vi "adc_avg.vi"(0 "CCS":T1={"Port Number"=1444, "Core Number"=1, "Page"=0}, 11 "error in":errorcluster) -> (4 "CCS out":T1={"Port Number"=1444, "Core Number"=1, "Page"=0})   [LabVIEW 2019]
uses:
  <userlib>/_TI-LA/Reusable/CCS/APIs/Data/Polymorphics/Write Data To Symbol - U16.vi
  <userlib>/_TI-LA/Reusable/CCS/APIs/Data/Polymorphics/Read Data From Symbol - U16 Array.vi
  <vilib>/Utility/file.llb/Write Delimited Spreadsheet (DBL).vi
  <vilib>/Utility/file.llb/Write Delimited Spreadsheet (I64).vi
  <userlib>/_TI-LA/Reusable/CCS/APIs/CCS.lvlib
panel:
  out "size(s)":i32
  out "x/y":dbl[](array[numeric])
  out "Array":i32[](array[numeric])
  out "error out":errorcluster
  # "uint16_t lv_ref_sel     =   0; //0=vdda, 1=extref, 2=intref\nuint16_t lv_ref_vol     =   0; //0=2P5V, 1=1P4V\nuint16_t lv_scomp       =   8; //8Clocks of 32M give = 250ns"
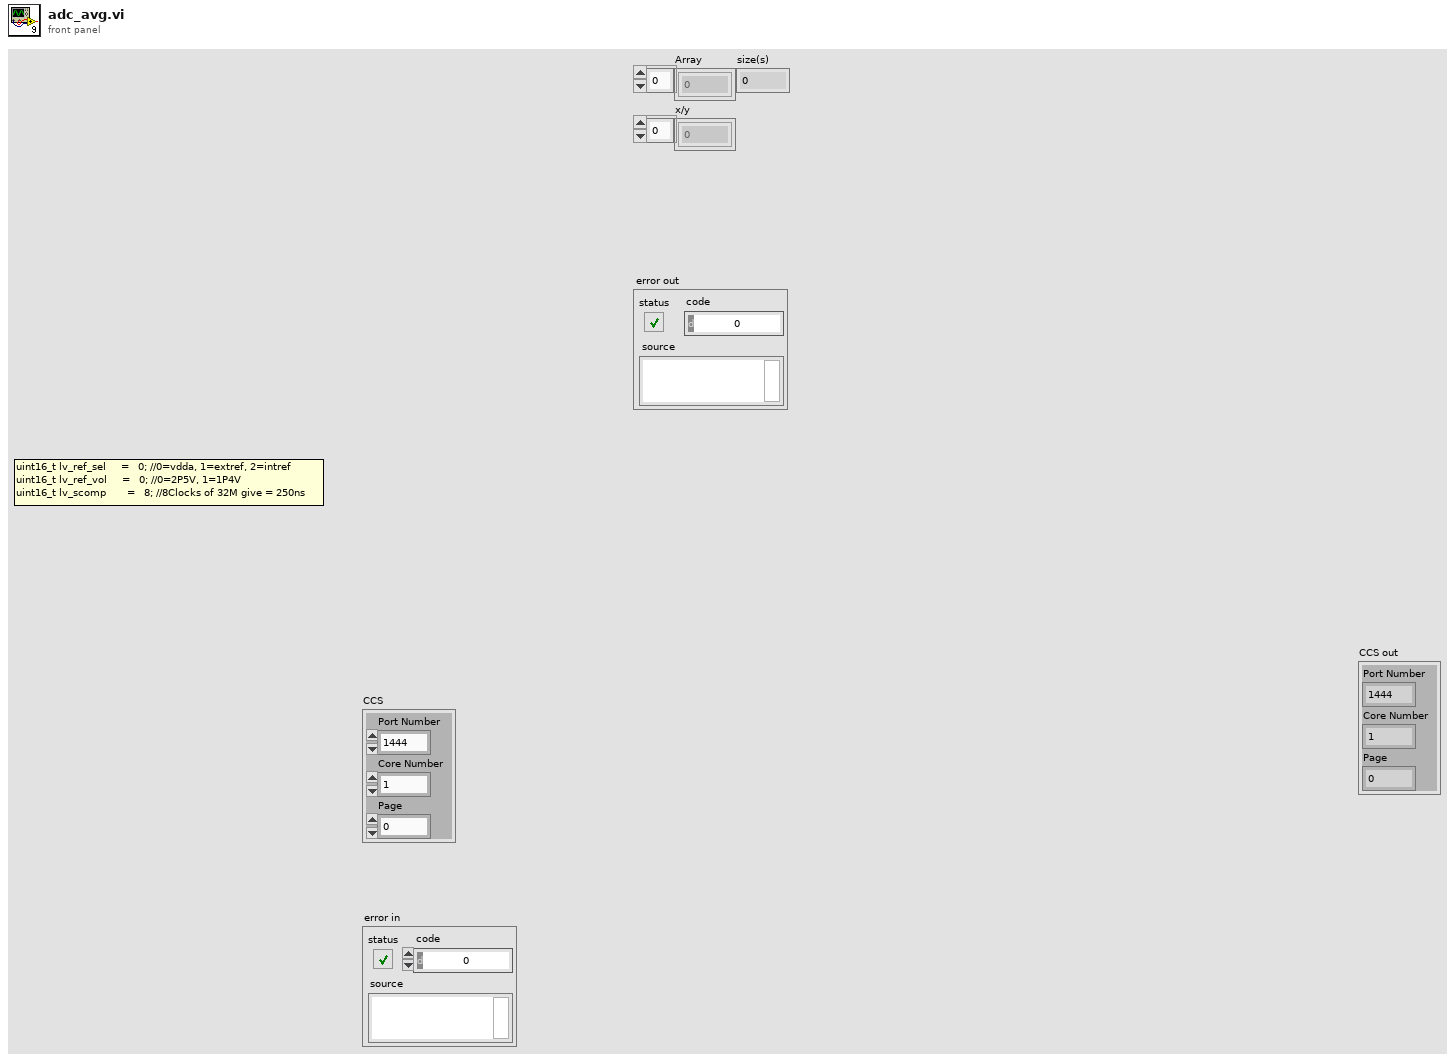
[diagram p1: front panel]
types:
  T1 = cluster{"Port Number":u16, "Core Number":u16, "Page":i32}
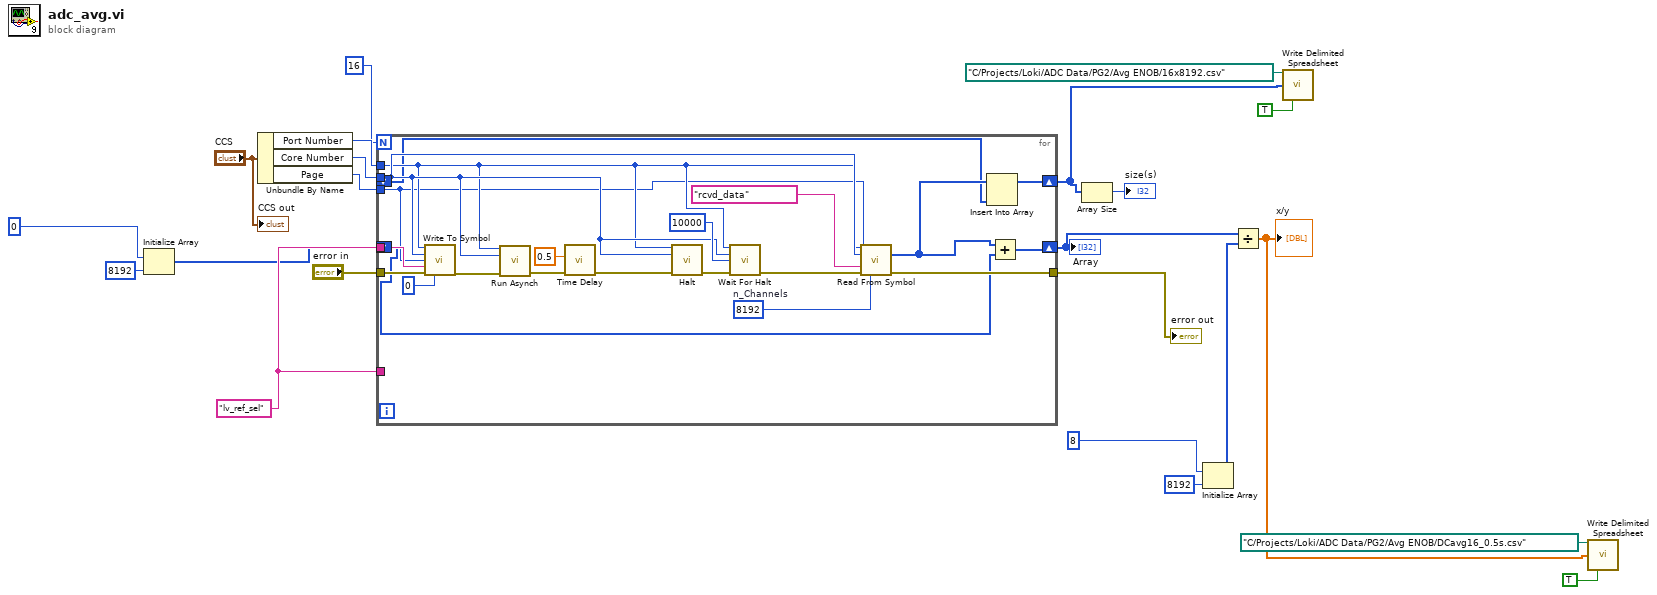
[diagram p0: block diagram]
diagram:
  w16 = "lv_ref_sel"
  n1 = Initialize Array(0, 8192 ("dimension size")) -> (w4:i32[])
  n2 = Unbundle By Name("CCS") -> ("Port Number"=w20:u16, "Core Number"=w18:u16, "Page"=w19:i32)
  n3 = for {
    N: 16 -> [_]
    tunnel: "error in" -> [w38]
    tunnel: w20 -> [w30]
    tunnel: w19 -> [w29]
    tunnel: w18 -> [w31]
    tunnel: w16 -> [w39]
    tunnel: w16 -> [_]
    tunnel: [w28] -> w15
    shift-right: [w27] -> w12
    shift-left: w4 -> [w25]
    shift-right: [w24] -> w1
    shift-left: _ -> [w23]
    w43 = u32 8192  # n_Channels
    n4 = call-poly <userlib>:"Write To Symbol.vi"("Port Number"=w30, "Core Number"=w31, "Page"=w29, "Symbol Name"=w39, "error in"=w38, "Write Data"=u16 0) -> ("error out"=w37:errorcluster)  [unwired: 7 in, 2 out]
    n5 = call <userlib>:"Run Asynch.vi"("Port Number"=w30, "Core Number"=w31, "error in"=w37) -> ("error out"=w36:errorcluster)  [unwired: 10 in, 2 out]
    n6 = call "Time Delay"("error in (no error)"=w36, "Delay Time (s)"=0.5) -> ("error out"=w35:errorcluster)  [unwired: 9 in]
    n7 = call <userlib>:"Halt.vi"("Port Number"=w30, "Core Number"=w31, "error in"=w35) -> ("error out"=w41:errorcluster)  [unwired: 10 in, 2 out]
    n8 = call <userlib>:"Wait For Halt.vi"("Port Number"=w30, "Core Number"=w31, "Timeout (10k)(ms)"=10000, "error in"=w41) -> ("error out"=w32:errorcluster)  [unwired: 9 in, 2 out]
    n9 = call-poly <userlib>:"Read From Symbol.vi"("Port Number"=w30, "Core Number"=w31, "Page"=w29, "Symbol Name"="rcvd_data", "error in"=w32, "Data Length"=w43) -> ("Read Data[]"=w26:u16[], "error out"=w28:errorcluster)  [unwired: 6 in, 2 out]
    n10 = Insert Into Array(array=w26, new element=w23) -> (w24:u16[])  [unwired: 1 in]
    n11 = Add(x=w26, y=w25) -> (x+y=w27:i32[])
  }
  "error out" <- w15
  "Array" <- w12
  n12 = Array Size(array=w1) -> (size(s)=→"size(s)":i32)
  n13 = Initialize Array(8, 8192 ("dimension size")) -> (w9:i32[])
  n14 = Divide(x=w12, y=w9) -> (x/y=w6:dbl[])
  "x/y" <- w6
  n15 = call-poly <vilib>:"Write Delimited Spreadsheet.vi"("file path (dialog if empty)"=path "C:/Projects/Loki/ADC Data/PG2/Avg ENOB/16x8192.csv", "1D data"=w1, "transpose? (no:F)"=TRUE) -> ()  [unwired: 11 in, 2 out]
  n16 = call-poly <vilib>:"Write Delimited Spreadsheet.vi"("file path (dialog if empty)"=path "C:/Projects/Loki/ADC Data/PG2/Avg ENOB/DCavg16_0.5s.csv", "1D data"=w6, "transpose? (no:F)"=TRUE) -> ()  [unwired: 11 in, 2 out]
  "CCS out" <- "CCS"
